vi "TPP-printer-v2.vi"() -> ()   [LabVIEW 2015]
uses:
  Kinesis/Thorlabs.MotionControl.Controls.dll
  <vilib>/DAQmx/write.llb/DAQmx Write (Digital Bool 1Line 1Point).vi
  <vilib>/Utility/file.llb/Read Delimited Spreadsheet (string).vi
  <vilib>/DAQmx/create/channels.llb/DAQmx Create Channel (DO-Digital Output).vi
  <vilib>/DAQmx/miscellaneous.llb/DAQmx Fill In Error Info.vi
panel:
  in  "物镜":u16(ring) items=["100X", "20X"]
  out "每层耗时/s":dbl
  out "每行耗时/s":dbl
  out "每点耗时/s":dbl
  in  "停止":bool
  in  "Z轴驱动序列号":string="27000001"
  in  "KCubeDCServoControl":refnum<k24>(container)
  in  "设定XY扫描速度(°/s)\n注：0代表最快速度":dbl
  out "当前G码":i32
  out "XYZ当前坐标":dbl[](array[numeric])
  in  "比例因子(V/°)":dbl=0.5
  in  "AO通道：X前Y后":tag="Dev1/ao0:1"
  out "当前扫描速度(°/s)":dbl
  in  "DO通道：shutter控制":tag="Dev1/port1/line0" caption="线"
  in  "导入TPP-code文件":path=path "C:/Users/Hongq/Desktop/grating切片2.txt"
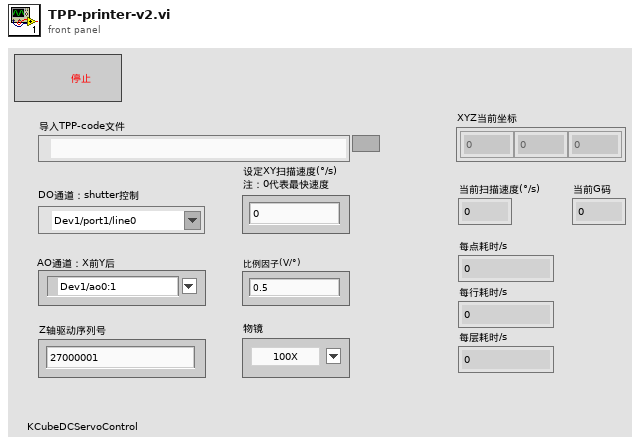
[diagram p1: front panel]
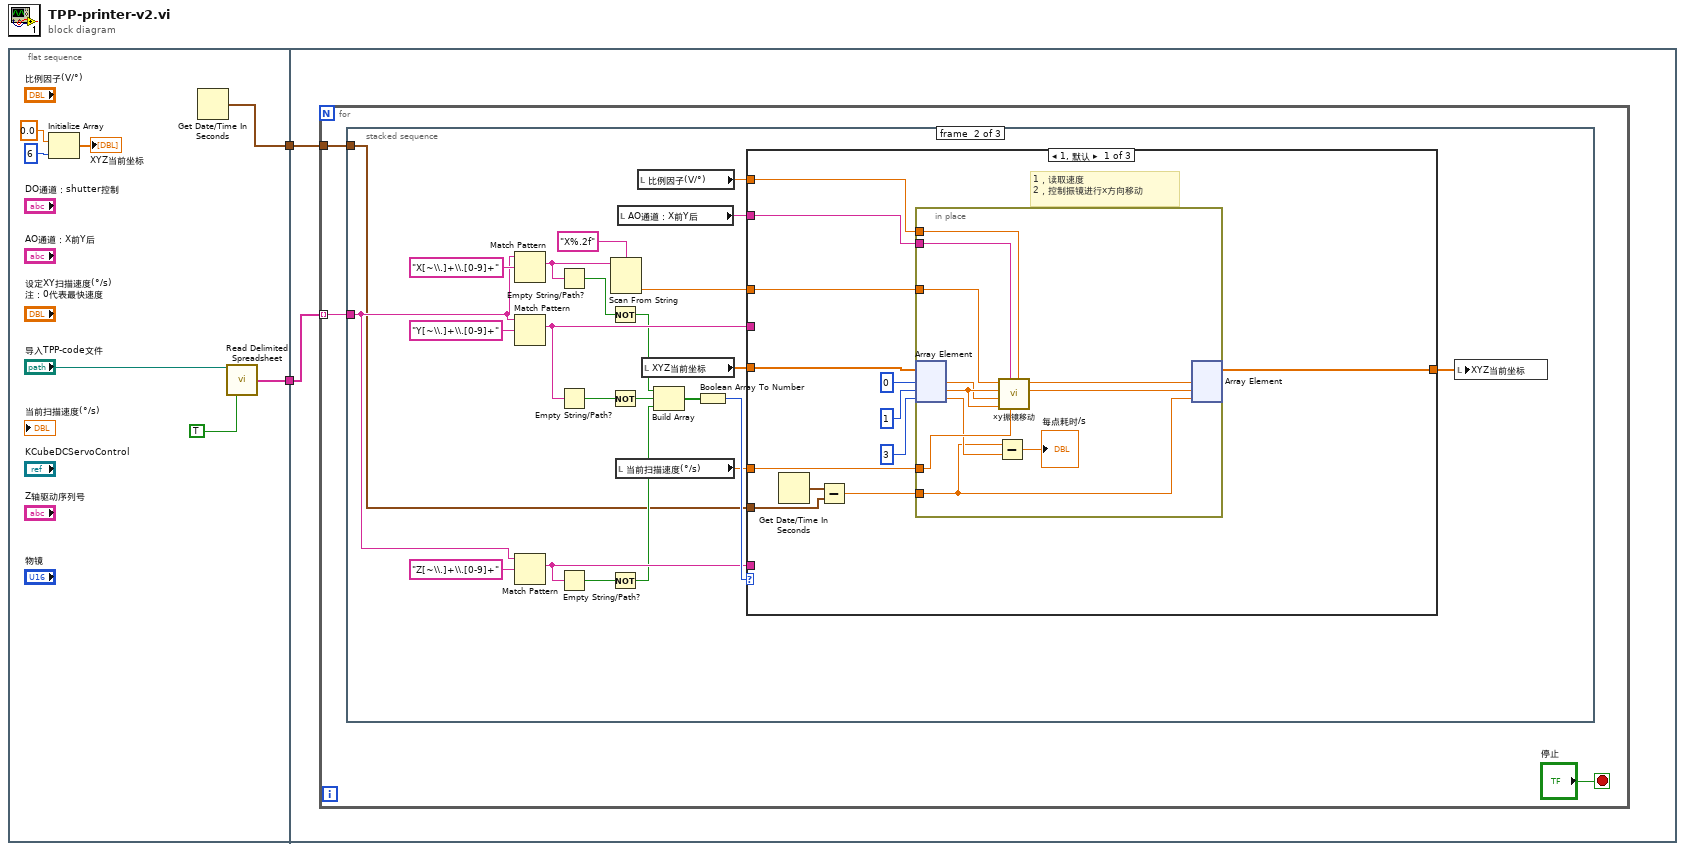
[diagram p0: block diagram]
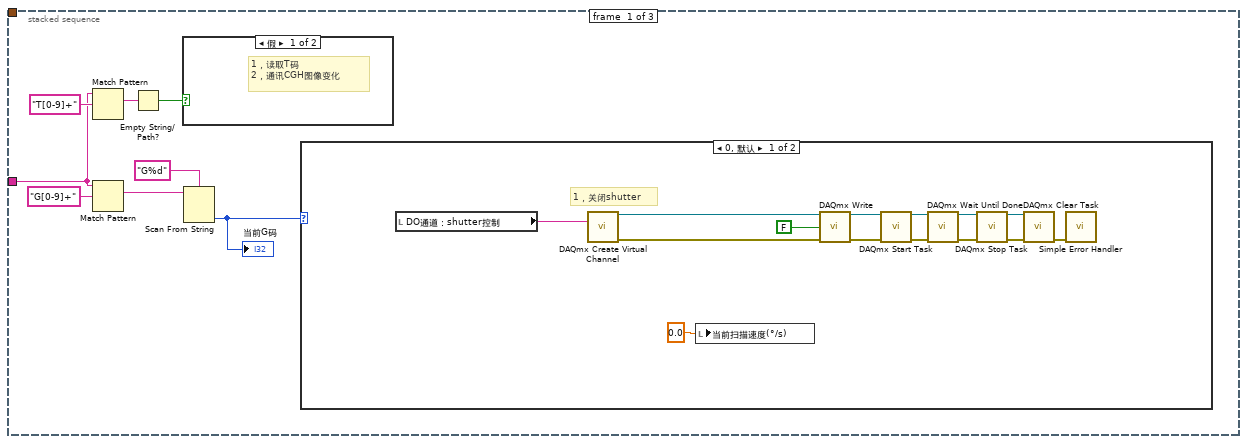
[diagram p2: hidden frame]
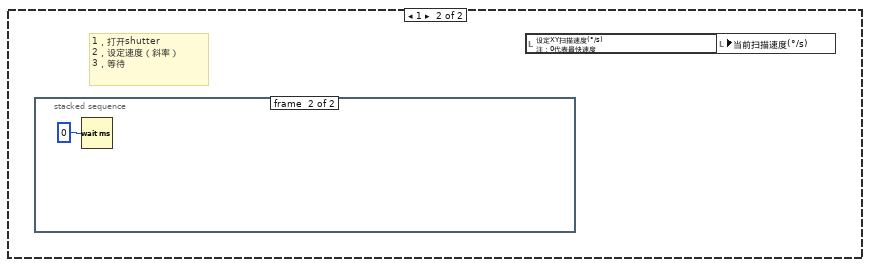
[diagram p4: hidden frame]
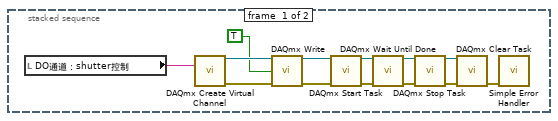
[diagram p5: hidden frame]
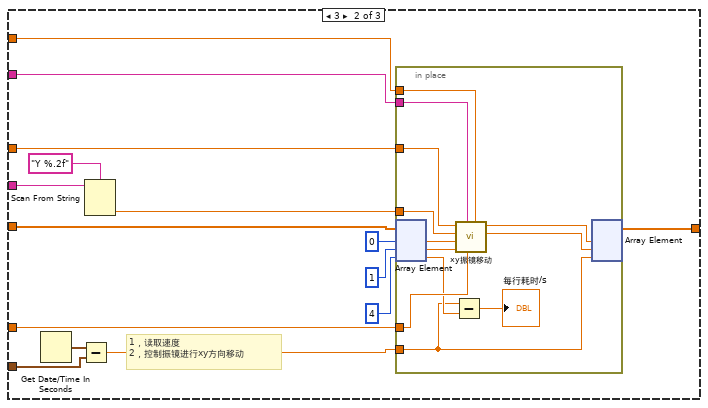
[diagram p6: hidden frame]
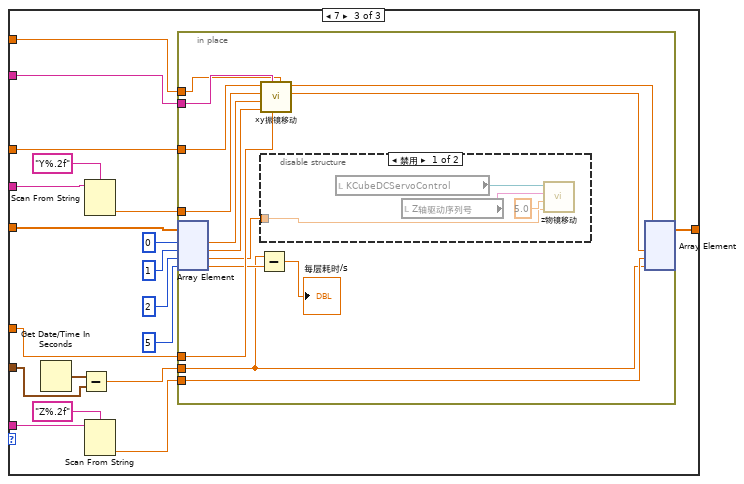
[diagram p7: hidden frame]
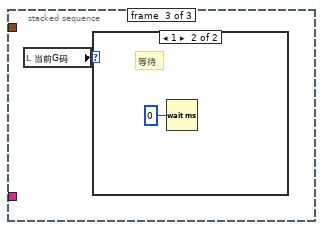
[diagram p9: hidden frame]
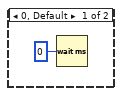
[diagram p10: hidden frame]
diagram:
  n1 = flat-sequence {
    tunnel: [w8] -> w2
    tunnel: [w3] -> w1
    tunnel: w2 -> [w11]
    tunnel: w1 -> [w10]
    frame #0 {
      n2 = Initialize Array(0.0 ("元素"), 6 ("维数大小")) -> (→"XYZ当前坐标":dbl[])
      n3 = Get Date/Time In Seconds() -> (seconds since 1Jan1904=w3:timestamp)
      n4 = call-poly <vilib>:"Read Delimited Spreadsheet.vi"("file path (dialog if empty)"="导入TPP-code文件", "transpose? (F)"=TRUE) -> ("first row"=w8:string[])  [unwired: 8 in, 5 out]
    }
    frame #1 {
      n5 = for {
        tunnel: w11 -> [w14] mode=indexing
        tunnel: w10 -> [w12]
        stop <- "停止" stop-if-true
        n6 = stacked-sequence {
          tunnel: w14 -> [w17 w71 _]
          tunnel: w12 -> [_ w52 _]
          frame #0 {
            n7 = Match Pattern(string=w17, regular expression="T[0-9]+" ("正则表达式")) -> (match substring=w18:string)  [unwired: 1 in, 3 out]
            n8 = Match Pattern(string=w17, regular expression="G[0-9]+" ("正则表达式")) -> (match substring=w20:string)  [unwired: 1 in, 3 out]
            n9 = Empty String/Path?(string/path=w18) -> (empty?=w16:bool)
            n10 = case shown="假" w16 {
              frame False {
                # "1，读取T码\n2，通讯CGH图像变化"
              }
              frame True {
                # "无处理"
              }
            }
            n11 = Scan From String(format string="G%d" ("格式字符串"), input string=w20) -> (output 1=w15:i32)  [unwired: 3 in, 3 out]
            "当前G码" <- w15
            n12 = case shown="0, 默认" w15 {
              frame 0, Default {
                # "1，关闭shutter"
                n13 = local read "DO通道：shutter控制"() -> (w24:tag)
                n14 = call-poly <vilib>:"DAQmx Create Virtual Channel.vi"("lines"=w24) -> ("task out"=w36:refnum<k21>, "error out"=w35:errorcluster)  [unwired: 13 in]
                n15 = local write "当前扫描速度(°/s)"(0.0 ("扫描速度(°/s)")) -> ()
                n16 = call-poly <vilib>:"DAQmx Write.vi"("task/channels in"=w36, "data"=FALSE, "error in"=w35) -> ("task out"=w33:refnum<k21>, "error out"=w32:errorcluster)  [unwired: 10 in, 1 out]
                n17 = call <vilib>:"DAQmx Start Task.vi"("task/channels in"=w33, "error in"=w32) -> ("task out"=w31:refnum<k21>, "error out"=w30:errorcluster)  [unwired: 12 in]
                n18 = call <vilib>:"DAQmx Wait Until Done.vi"("task/channels in"=w31, "error in"=w30) -> ("task out"=w29:refnum<k21>, "error out"=w28:errorcluster)  [unwired: 12 in]
                n19 = call <vilib>:"DAQmx Stop Task.vi"("task/channels in"=w29, "error in"=w28) -> ("task out"=w27:refnum<k21>, "error out"=w26:errorcluster)  [unwired: 12 in]
                n20 = call <vilib>:"DAQmx Clear Task.vi"("task in"=w27, "error in"=w26) -> ("error out"=w25:errorcluster)  [unwired: 13 in]
                n21 = call <vilib>:"Simple Error Handler.vi"("error in (no error)"=w25) -> ()  [unwired: 4 in, 5 out]
              }
              frame 1 {
                # "1，打开shutter\n2，设定速度（斜率）\n3，等待"
                n22 = stacked-sequence {
                  frame #0 {
                    n23 = local read "DO通道：shutter控制"() -> (w38:tag)
                    n24 = call-poly <vilib>:"DAQmx Create Virtual Channel.vi"("lines"=w38) -> ("task out"=w50:refnum<k21>, "error out"=w49:errorcluster)  [unwired: 13 in]
                    n25 = call-poly <vilib>:"DAQmx Write.vi"("task/channels in"=w50, "data"=TRUE, "error in"=w49) -> ("task out"=w47:refnum<k21>, "error out"=w46:errorcluster)  [unwired: 10 in, 1 out]
                    n26 = call <vilib>:"DAQmx Start Task.vi"("task/channels in"=w47, "error in"=w46) -> ("task out"=w45:refnum<k21>, "error out"=w44:errorcluster)  [unwired: 12 in]
                    n27 = call <vilib>:"DAQmx Wait Until Done.vi"("task/channels in"=w45, "error in"=w44) -> ("task out"=w43:refnum<k21>, "error out"=w42:errorcluster)  [unwired: 12 in]
                    n28 = call <vilib>:"DAQmx Stop Task.vi"("task/channels in"=w43, "error in"=w42) -> ("task out"=w41:refnum<k21>, "error out"=w40:errorcluster)  [unwired: 12 in]
                    n29 = call <vilib>:"DAQmx Clear Task.vi"("task in"=w41, "error in"=w40) -> ("error out"=w39:errorcluster)  [unwired: 13 in]
                    n30 = call <vilib>:"Simple Error Handler.vi"("error in (no error)"=w39) -> ()  [unwired: 4 in, 5 out]
                  }
                  frame #1 {
                    n31 = Wait (ms)(milliseconds to wait=u32 0 ("等待时间（毫秒）")) -> ()  [unwired: 1 out]
                  }
                }
                n32 = local read "设定XY扫描速度(°/s)\n注：0代表最快速度"() -> (w37:dbl)
                n33 = local write "当前扫描速度(°/s)"(w37) -> ()
              }
            }
          }
          frame #1 {
            n34 = Match Pattern(string=w71, regular expression="X[~\\.]+\\.[0-9]+" ("正则表达式")) -> (match substring=w65:string)  [unwired: 1 in, 3 out]
            n35 = Match Pattern(string=w71, regular expression="Y[~\\.]+\\.[0-9]+" ("正则表达式")) -> (match substring=w68:string)  [unwired: 1 in, 3 out]
            n36 = Match Pattern(string=w71, regular expression="Z[~\\.]+\\.[0-9]+" ("正则表达式")) -> (match substring=w67:string)  [unwired: 1 in, 3 out]
            n37 = Empty String/Path?(string/path=w65) -> (empty?=w58:bool)
            n38 = Empty String/Path?(string/path=w68) -> (empty?=w57:bool)
            n39 = Empty String/Path?(string/path=w67) -> (empty?=w55:bool)
            n40 = Not(x=w58) -> (.not. x?=w53:bool)
            n41 = Not(x=w57) -> (.not. x?=w56:bool)
            n42 = Not(x=w55) -> (.not. x?=w54:bool)
            n43 = Scan From String(format string="X%.2f" ("格式字符串"), input string=w65) -> (output 1=w64:dbl)  [unwired: 3 in, 3 out]
            n44 = local read "当前扫描速度(°/s)"() -> (w61:dbl)
            n45 = local read "AO通道：X前Y后"() -> (w59:tag)
            n46 = local read "比例因子(V/°)"() -> (w60:dbl)
            n47 = local read "XYZ当前坐标"() -> (w63:dbl[])
            n48 = Build Array(w53, w56, w54) -> (w70:bool[])
            n49 = Boolean Array To Number(Boolean array=w70) -> (number=w69:u32)
            n50 = case shown="1, 默认" w69 {
              tunnel: w68 -> [_ w112 w137]
              tunnel: w67 -> [_ _ w130]
              tunnel: w59 -> [w80 w103 w138]
              tunnel: w60 -> [w79 w102 w139]
              tunnel: w64 -> [w82 w105 w136]
              tunnel: w63 -> [w86 w107 w135]
              tunnel: [w85 w106 w132] -> w62
              tunnel: w61 -> [w81 w108 w134]
              tunnel: w52 -> [w77 w100 w127]
              frame 1, Default {
                # "1，读取速度\n2，控制振镜进行x方向移动"
                n51 = Get Date/Time In Seconds() -> (seconds since 1Jan1904=w78:timestamp)
                n52 = Subtract(x=w78, y=w77) -> (x-y=w75:dbl)
                n53 = in-place {
                  in-place-border: w82 -> [w95]
                  in-place-border: w81 -> [w94]
                  in-place-border: w80 -> [w93]
                  in-place-border: w79 -> [w92]
                  in-place-border: w75 -> [w87]
                  n54 = in-place-array #1(w86, 0, 1, 3) -> (w96:dbl, w97:dbl, w89:dbl)
                  n55 = Subtract(x=w87, y=w89) -> (x-y=→"每点耗时/s":dbl)
                  n56 = call "xy振镜移动.vi"("比例因子(V/°)"=w92, "速度(°/s)"=w94, "AO通道：X前Y后"=w93, "Y初始角(°)"=w97, "X初始角(°)"=w96, "Y终止角(°)"=w97, "X终止角(°)"=w95) -> ("Y终止角(°) 2"=w90:dbl, "X终止角(°) 2"=w91:dbl)  [unwired: 2 in]
                  n57 = in-place-array #1(w91, w90, w87) -> (w85:dbl[])  [unwired: 3 out]
                }
              }
              frame 3 {
                # "1，读取速度\n2，控制振镜进行xy方向移动"
                n58 = Get Date/Time In Seconds() -> (seconds since 1Jan1904=w101:timestamp)
                n59 = Subtract(x=w101, y=w100) -> (x-y=w98:dbl)
                n60 = Scan From String(format string="Y %.2f" ("格式字符串"), input string=w112) -> (output 1=w104:dbl)  [unwired: 3 in, 3 out]
                n61 = in-place {
                  in-place-border: w105 -> [w122]
                  in-place-border: w108 -> [w121]
                  in-place-border: w103 -> [w120]
                  in-place-border: w102 -> [w119]
                  in-place-border: w104 -> [w116]
                  in-place-border: w98 -> [w113]
                  n62 = in-place-array #2(w107, 0, 1, 4) -> (w123:dbl, w124:dbl, w115:dbl)
                  n63 = Subtract(x=w113, y=w115) -> (x-y=→"每行耗时/s":dbl)
                  n64 = call "xy振镜移动.vi"("比例因子(V/°)"=w119, "速度(°/s)"=w121, "AO通道：X前Y后"=w120, "Y初始角(°)"=w124, "X初始角(°)"=w123, "Y终止角(°)"=w116, "X终止角(°)"=w122) -> ("Y终止角(°) 2"=w117:dbl, "X终止角(°) 2"=w118:dbl)  [unwired: 2 in]
                  n65 = in-place-array #2(w118, w117, w113) -> (w106:dbl[])  [unwired: 3 out]
                }
              }
              frame 7 {
                n66 = Get Date/Time In Seconds() -> (seconds since 1Jan1904=w128:timestamp)
                n67 = Subtract(x=w128, y=w127) -> (x-y=w125:dbl)
                n68 = Scan From String(format string="Y%.2f" ("格式字符串"), input string=w137) -> (output 1=w143:dbl)  [unwired: 3 in, 3 out]
                n69 = Scan From String(format string="Z%.2f" ("格式字符串"), input string=w130) -> (output 1=w129:dbl)  [unwired: 3 in, 3 out]
                n70 = in-place {
                  in-place-border: w136 -> [w155]
                  in-place-border: w134 -> [w154]
                  in-place-border: w138 -> [w153]
                  in-place-border: w139 -> [w152]
                  in-place-border: w143 -> [w149]
                  in-place-border: w129 -> [w147]
                  in-place-border: w125 -> [w144]
                  n71 = in-place-array #3(w135, 0, 1, 2, 5) -> (w156:dbl, w157:dbl, w148:dbl, w146:dbl)
                  n72 = Subtract(x=w144, y=w146) -> (x-y=→"每层耗时/s":dbl)
                  n73 = call "xy振镜移动.vi"("比例因子(V/°)"=w152, "速度(°/s)"=w154, "AO通道：X前Y后"=w153, "Y初始角(°)"=w157, "X初始角(°)"=w156, "Y终止角(°)"=w149, "X终止角(°)"=w155) -> ("Y终止角(°) 2"=w150:dbl, "X终止角(°) 2"=w151:dbl)  [unwired: 2 in]
                  n74 = disable-structure shown="禁用" {
                    disable-tunnel: w148 -> [w158 _]
                    frame Disabled {
                      n75 = local read "KCubeDCServoControl"() -> (w161:refnum<k24>)
                      n76 = local read "Z轴驱动序列号"() -> (w160:string)
                      n77 = call "z物镜移动.vi"("position"=w158, "maxVelocity"=5.0, "SerialNumber"=w160, "KCubeDCServoControl"=w161) -> ()  [unwired: 5 in, 3 out]
                    }
                    frame Enabled {
                    }
                  }
                  n78 = in-place-array #3(w151, w150, w147, w144) -> (w132:dbl[])  [unwired: 4 out]
                }
              }
            }
            n79 = local write "XYZ当前坐标"(w62) -> ()
          }
          frame #2 {
            n80 = local read "当前G码"() -> (w162:i32)
            n81 = case shown="1" w162 {
              frame 0, Default {
                n82 = Wait (ms)(milliseconds to wait=u32 0 ("等待时间（毫秒）")) -> ()  [unwired: 1 out]
              }
              frame 1 {
                # "等待"
                n83 = Wait (ms)(milliseconds to wait=u32 0 ("等待时间（毫秒）")) -> ()  [unwired: 1 out]
              }
            }
          }
        }
      }
    }
  }
